vi "write_swabian_ht3v2_header.vi"(0 "data_path":path, 1 "acq_time":i32, 2 "sync_rate":i32, 3 "acq_mode":i32, 5 "data_comment":string, 7 "num_records":u64, 11 "error in (no error)":errorcluster) -> (15 "error out":errorcluster)   [LabVIEW 2018]
uses:
  cmake-build-release/swabian_lib.dll
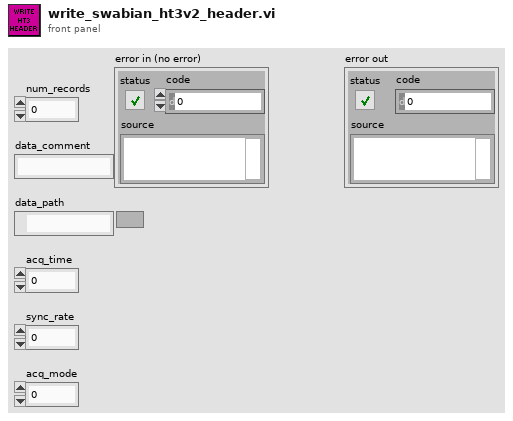
[diagram p1: front panel]
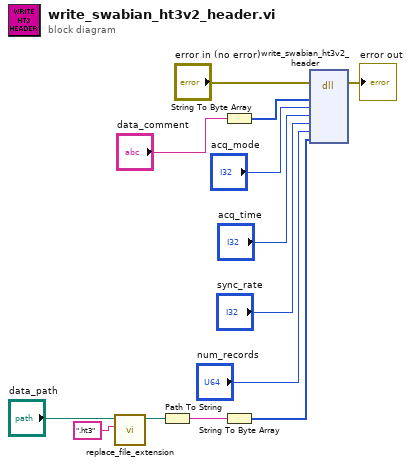
[diagram p0: block diagram]
diagram:
  n1 = call "replace_file_extension.vi"("new_extension"=".ht3", "data_path"="data_path") -> ("appended path"=w5:path)  [unwired: 8 in, 1 out]
  n2 = Path To String(path=w5) -> (string=w12:string)
  n3 = String To Byte Array(string="data_comment") -> (unsigned byte array=w11:u8[])
  n4 = String To Byte Array(string=w12) -> (unsigned byte array=w13:u8[])
  n5 = dll-call lib="C:/Users/bspoka/Documents/swabian_LV/swabian_vis/swabian_lib/cmake-build-release/swabian_lib.dll" fn="write_swabian_ht3v2_header"(error in="error in (no error)", "data_comment"=w11, "acq_mode"="acq_mode", "acq_time"="acq_time", "sync_rate"="sync_rate", "num_records"="num_records", "data_path"=w13) -> (error out=→"error out":errorcluster)  [unwired: 9 in, 1 out]
